vi "Read_Spreadsheet.vi"() -> (3 "Data In":T1)   [LabVIEW 2017]
doc: "Leer spreadsheet para obtener los valores del documento."
uses:
  Controls/Data_In.ctl
  <vilib>/Utility/file.llb/Read Delimited Spreadsheet (string).vi
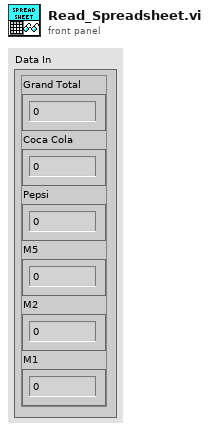
[diagram p1: front panel]
types:
  T1 = typedef "Data_In.ctl" = cluster{"Grand Total":i32, "Coca Cola":i32, "Pepsi":i32, "M5":i32, "M2":i32, "M1":i32}
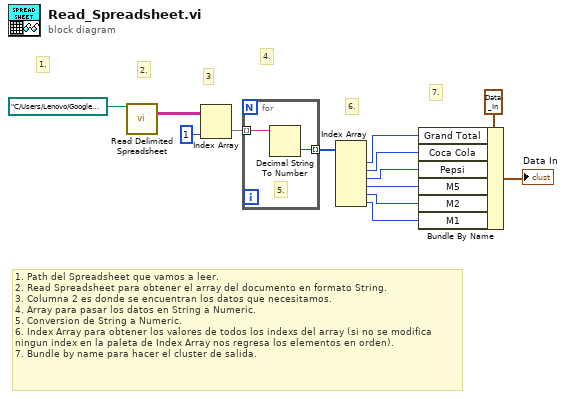
[diagram p0: block diagram]
diagram:
  # "1. Path del Spreadsheet que vamos a leer.\n2. Read Spreadsheet para obtener el array del documento en formato String.\n3. Columna 2 es donde se encuentran los datos que necesitamos.\n4. Array para pasar los datos en String a Numeric.\n5. Conversion de String a Numeric.\n6. Index Array para obtener los valores de todos los indexs del array (si no se modifica\nningun index en la paleta de Index Array nos regresa los elementos en orden).\n7. Bundle by name para hacer el cluster de salida."
  # "7."
  # "6."
  # "4."
  # "3"
  # "2."
  # "1."
  n1 = call-poly <vilib>:"Read Delimited Spreadsheet.vi"("file path (dialog if empty)"=path "C:/Users/Lenovo/Google Drive/Labview/Curso (FIME)/HW/Act. 3/HW. 3/Stuff/Data.txt") -> ("all rows"=w12:string[][])  [unwired: 9 in, 5 out]
  n2 = Index Array(array=w12, index (col)=1 ("disabled index (col)")) -> (element=w10:string[])  [unwired: 1 in]
  n3 = for {
    tunnel: w10 -> [w15] mode=indexing
    tunnel: [w14] -> w9 mode=indexing
    # "5."
    n4 = Decimal String To Number(string=w15) -> (number=w14:i32)  [unwired: 2 in, 1 out]
  }
  n5 = Index Array(array=w9) -> (element #1=w7:i32, element #2=w6:i32, element #3=w5:i32, element #4=w4:i32, element #5=w3:i32, element #6=w2:i32)  [unwired: 6 in]
  n6 = Bundle By Name(cluster=T1 {"Grand Total"=0, "Coca Cola"=0, "Pepsi"=0, "M5"=0, "M2"=0, "M1"=0} ("Data In"), "Grand Total"=w7, "Coca Cola"=w6, "Pepsi"=w5, "M5"=w4, "M2"=w3, "M1"=w2) -> (→"Data In":T1)
